vi "Keithley 2410 Set Voltage and Measure Current.vi"(6 "milliseconds to wait":u32=50, 7 "Source Mode  (0: Voltage)":u16(ring) items=["Voltage", "Current"], 8 "Compliance  Level (1uA)":dbl=1e-06, 9 "Number of Samples":u32=5, 10 "Source Value (Volts or Amps)":dbl=0.2, 11 "VISA resource name":refnum<visa-resource-name>="GPIB0::24::INSTR") -> (0 "mean resistence":dbl format="%0.5e", 1 "standard deviation current measured":dbl format="%0.5e", 2 "mean current measured":dbl format="%0.5e", 3 "standard deviation of voltage applied":dbl format="%0.2f", 4 "standard deviation of resistance":dbl format="%0.5e", 5 "Mean Voltage Applied":dbl format="%0.2f")   [LabVIEW 2023]
doc: "Configures a sweep and takes voltage and current readings at each point."
uses:
  <instrlib>/Keithley 24XX/Public/Data/Read (Multiple Points).vi
  <instrlib>/Keithley 24XX/Keithley 24XX.lvlib
  <vilib>/Analysis/NI_AALBase.lvlib
panel:
  in  "Serial Configuration":T1={"Baud Rate"=9600, "Parity"=0, "Data Bits"=8, "Stop Bits"=10, "Flow Control"=0} {"Flow Control" items=["None", "XON/XOFF", "RTS/CTS", "XON/XOFF & RTS/CTS", "DTR/DSR", "XON/XOFF & DTR/DSR"]; "Stop Bits" items=["1.0"=10, "1.5"=15, "2.0"=20]; "Data Bits" items=["7"=7, "8"=8]; "Parity" items=["None", "Odd", "Even", "Mark", "Space"]; "Baud Rate" items=["300"=300, "600"=600, "1200"=1200, "2400"=2400, "4800"=4800, "9600"=9600, "19200"=19200]}
  # "Keithley 2410-C Set and Measure"
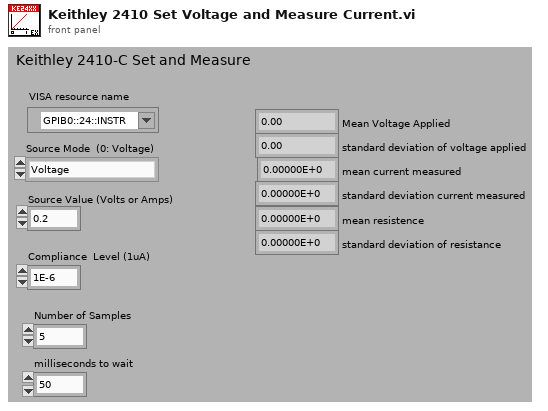
[diagram p1: front panel]
types:
  T1 = cluster{"Baud Rate":u32, "Parity":u16, "Data Bits":u16, "Stop Bits":u16, "Flow Control":u16}
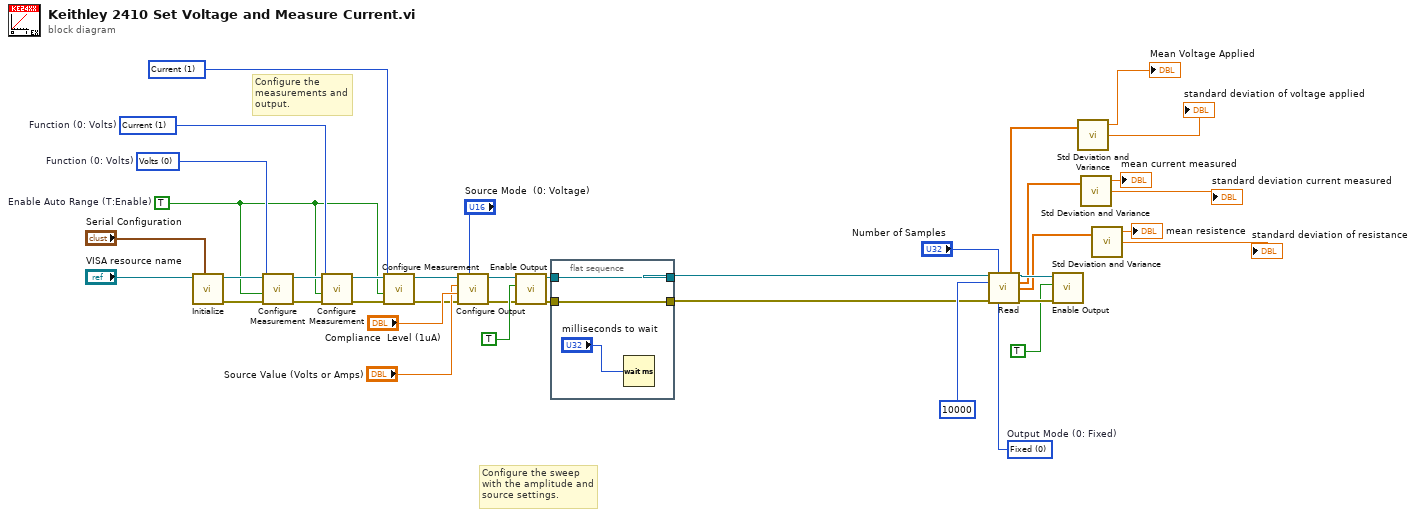
[diagram p0: block diagram]
diagram:
  w1 = u16 1 items=["Volts", "Current", "Resistance"] ("Function (0: Volts)")
  w2 = TRUE  # Enable Auto Range (T:Enable)
  w26 = u16 1 items=["Volts", "Current", "Resistance"]  # Function (0: Volts)
  w27 = u16 0 items=["Volts", "Current", "Resistance"]  # Function (0: Volts)
  w31 = u16 0 items=["Fixed", "Sweep", "List"]  # Output Mode (0: Fixed)
  # "Configure the sweep with the amplitude and source settings."
  # "Configure the measurements and output."
  n1 = call <instrlib>:"Initialize.vi"("Serial Configuration"="Serial Configuration", "VISA resource name"="VISA resource name") -> ("error out"=w38:errorcluster, "VISA resource name out"=w39:refnum<visa-resource-name>)  [unwired: 8 in]
  n2 = call <instrlib>:"Configure Measurement.vi"("error in (no error)"=w38, "Enable Auto Range (T:Enable)"=w2, "Function (0: Volts)"=w27, "VISA resource name"=w39) -> ("error out"=w37:errorcluster, "VISA resource name out"=w36:refnum<visa-resource-name>)  [unwired: 6 in]
  n3 = call <instrlib>:"Configure Measurement.vi"("error in (no error)"=w37, "Enable Auto Range (T:Enable)"=w2, "Function (0: Volts)"=w26, "VISA resource name"=w36) -> ("error out"=w3:errorcluster, "VISA resource name out"=w6:refnum<visa-resource-name>)  [unwired: 6 in]
  n4 = call <instrlib>:"Configure Measurement.vi"("error in (no error)"=w3, "Enable Auto Range (T:Enable)"=w2, "Function (0: Volts)"=w1, "VISA resource name"=w6) -> ("error out"=w4:errorcluster, "VISA resource name out"=w5:refnum<visa-resource-name>)  [unwired: 6 in]
  n5 = call <instrlib>:"Configure Output.vi"("Source Mode  (0: Voltage)"="Source Mode  (0: Voltage)", "error in (no error)"=w4, "Compliance  Level (0.1)"="Compliance  Level (1uA)", "Output Level (0)"="Source Value (Volts or Amps)", "VISA resource name"=w5) -> ("error out"=w22:errorcluster, "VISA resource name out"=w23:refnum<visa-resource-name>)  [unwired: 5 in]
  n6 = call <instrlib>:"Enable Output.vi"("error in (no error)"=w22, "Enable Output (T: Enable)"=TRUE, "VISA resource name"=w23) -> ("error out"=w19:errorcluster, "VISA resource name out"=w17:refnum<visa-resource-name>)  [unwired: 7 in]
  n7 = flat-sequence {
    tunnel: w19 -> [w42]
    tunnel: [w42] -> w18
    tunnel: w17 -> [w41]
    tunnel: [w41] -> w16
    frame #0 {
      n8 = Wait (ms)(milliseconds to wait="milliseconds to wait") -> ()  [unwired: 1 out]
    }
  }
  n9 = call-poly <instrlib>:"Read.vi"("VISA resource name"=w16, "Sample Count (1)"="Number of Samples", "Timeout (10000 ms)"=10000, "error in (no error)"=w18, "Output Mode (0: Fixed)"=w31) -> ("Voltage"=w15:sgl[], "VISA resource name out"=w29:refnum<visa-resource-name>, "Current"=w14:sgl[], "Resistance"=w9:sgl[], "error out"=w30:errorcluster)  [unwired: 4 in, 2 out]
  n10 = call <instrlib>:"Enable Output.vi"("error in (no error)"=w30, "Enable Output (T: Enable)"=TRUE, "VISA resource name"=w29) -> ()  [unwired: 7 in, 2 out]
  n11 = call <vilib>:"Std Deviation and Variance.vi"("X"=w15) -> ("mean"=→"Mean Voltage Applied":dbl, "standard deviation"=→"standard deviation of voltage applied":dbl)  [unwired: 1 in, 1 out]
  n12 = call <vilib>:"Std Deviation and Variance.vi"("X"=w14) -> ("mean"=→"mean current measured":dbl, "standard deviation"=→"standard deviation current measured":dbl)  [unwired: 1 in, 1 out]
  n13 = call <vilib>:"Std Deviation and Variance.vi"("X"=w9) -> ("mean"=→"mean resistence":dbl, "standard deviation"=→"standard deviation of resistance":dbl)  [unwired: 1 in, 1 out]
